vi "Test Setting.vi"   [LabVIEW 2020]
uses:
  Views/Setting View/Setting View/Setting View.lvclass
  C:/Program Files (x86)/National Instruments/LabVIEW 2020/vi.lib/ActorFramework/Actor/Actor.lvclass
  <vilib>/ActorFramework/Message Enqueuer/Message Enqueuer.lvclass/Message Enqueuer.ctl
  <vilib>/ActorFramework/Message Enqueuer/Enqueue.vi
  Depden On/Abstruct View/Abstruct View Messages/Show Front Msg/Show Front Msg.lvclass
  C:/Program Files (x86)/National Instruments/LabVIEW 2020/vi.lib/ActorFramework/Message/Message.lvclass
  <vilib>/ActorFramework/Message Priority Queue/Priority Enqueue.vi
  <vilib>/ActorFramework/Actor/Actor.lvclass
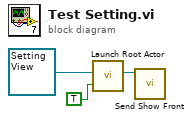
[diagram p0: block diagram]
diagram:
  n1 = call <vilib>:"Launch Root Actor.vi"("Open Actor Core front panel? (F)"=TRUE, "Actor"=refnum<class "Setting View.lvclass"> refnum ("[V]Setting View.lvlib:Setting View.lvclass")) -> ("Actor's Enqueuer"=w2:refnum<class "Message Enqueuer.lvclass">)  [unwired: 8 in, 1 out]
  n2 = call "Send Show Front.vi"("Message Enqueuer"=w2) -> ()  [unwired: 9 in, 2 out]
